vi "Expand.vi"(8 "error in (no error)":errorcluster, 9 "CurrentLinkedNodes":refnum<data-value>[](array[refnum]), 10 "NodeToExpand in":refnum<data-value>, 11 "OccupancyMap in":refnum<class "OccupancyMap.lvclass">) -> (0 "error out":errorcluster, 1 "NodesToLinkAndExpand":refnum<data-value>[](array[refnum]), 2 "NodeToExpand out":refnum<data-value>, 3 "OccupancyMap out":refnum<class "OccupancyMap.lvclass">)   [LabVIEW 2010, in "OccupancyMap.lvclass"]
uses:
  OccupancyMap.lvclass
  GraphNode/GraphNode.lvclass
  Cell/Cell.lvclass
  OccupancyMap.lvclass/OccupancyMap.ctl
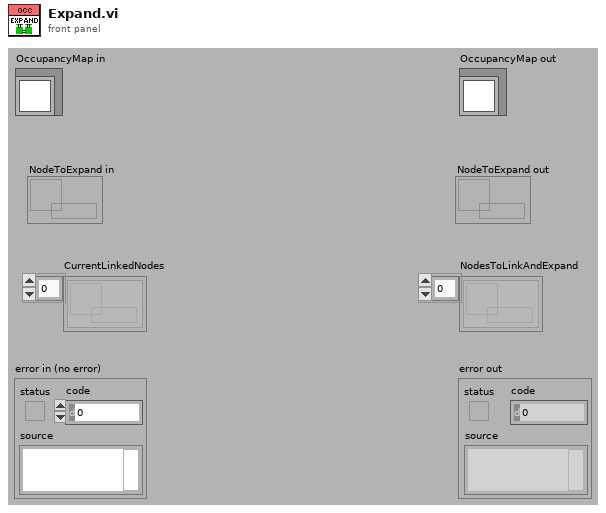
[diagram p1: front panel]
types:
  T1 = cluster{"Left":dbl, "Right":dbl, "Top":dbl, "Bottom":dbl}
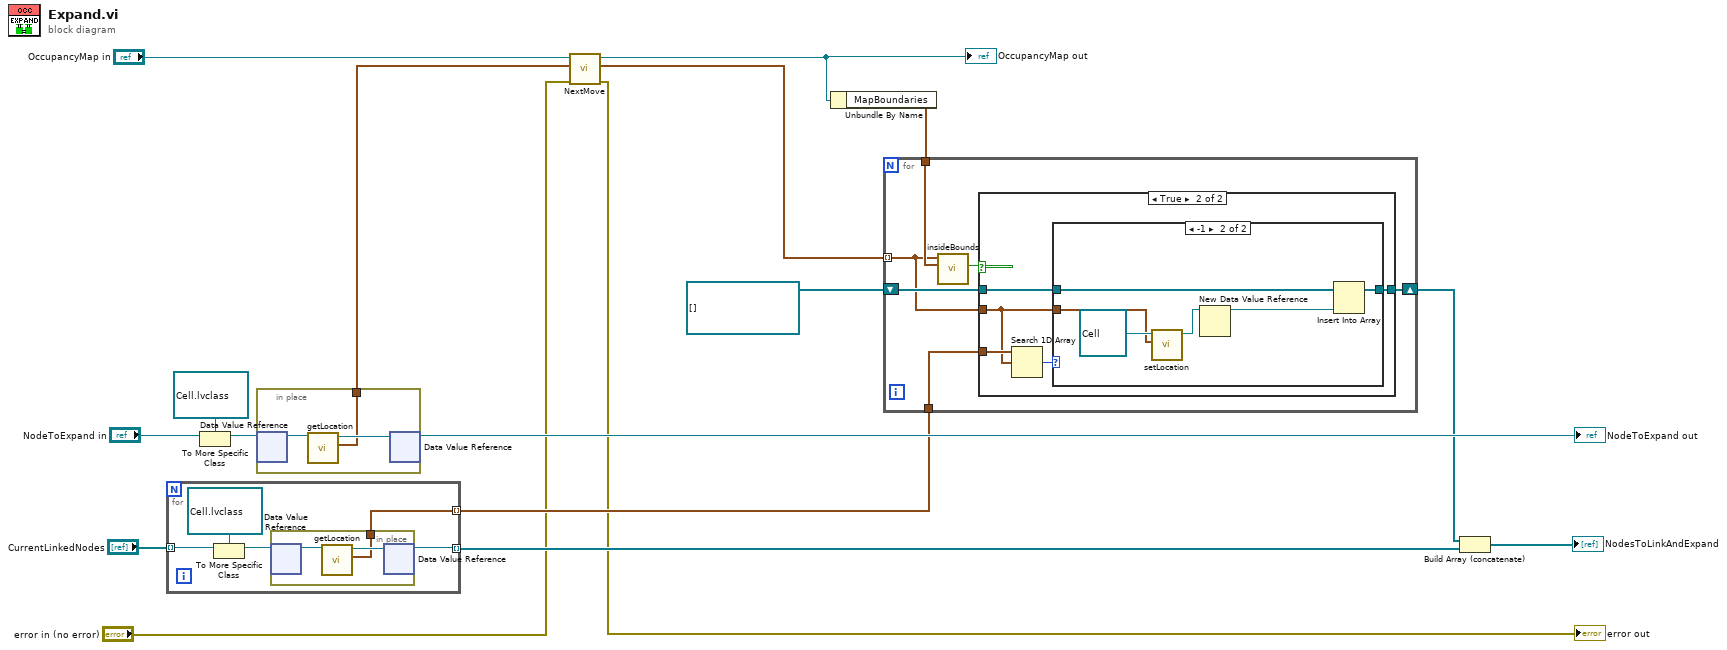
[diagram p0: block diagram]
diagram:
  n1 = for {
    tunnel: "CurrentLinkedNodes" -> [w20] mode=indexing
    tunnel: [w19] -> w11 mode=indexing
    tunnel: [w18] -> w8 mode=indexing
    n2 = To More Specific Class(target class=refnum<data-value> refnum ("data value reference"), reference=w20) -> (specific class reference=w22:refnum<data-value>)  [unwired: 1 in, 1 out]
    n3 = in-place {
      in-place-border: [w23] -> w19
      n4 = in-place-dvr #1(w22) -> (w25:refnum<class "Cell.lvclass">)  [unwired: 1 out]
      n5 = call "getLocation.vi"("Cell in"=w25) -> ("Location"=w23:cluster{"X":dbl, "Y":dbl}, "Cell out"=w24:refnum<class "Cell.lvclass">)  [unwired: 8 in, 1 out]
      n6 = in-place-dvr #1(w24) -> (w18:refnum<data-value>)  [unwired: 1 out]
    }
  }
  n7 = To More Specific Class(target class=refnum<data-value> refnum ("data value reference"), reference="NodeToExpand in") -> (specific class reference=w15:refnum<data-value>)  [unwired: 1 in, 1 out]
  n8 = in-place {
    in-place-border: [w26] -> w2
    n9 = in-place-dvr #2(w15) -> (w28:refnum<class "Cell.lvclass">)  [unwired: 1 out]
    n10 = call "getLocation.vi"("Cell in"=w28) -> ("Location"=w26:cluster{"X":dbl, "Y":dbl}, "Cell out"=w27:refnum<class "Cell.lvclass">)  [unwired: 8 in, 1 out]
    n11 = in-place-dvr #2(w27) -> (→"NodeToExpand out":refnum<data-value>)  [unwired: 1 out]
  }
  n12 = call "NextMove.vi"("error in (no error)"="error in (no error)", "Point"=w2, "OccupancyMap in"="OccupancyMap in") -> ("error out"=→"error out":errorcluster, "NextMove"=w1:cluster{"X":dbl, "Y":dbl}[], "OccupancyMap out"=w5:refnum<class "OccupancyMap.lvclass">)  [unwired: 6 in]
  "OccupancyMap out" <- w5
  n13 = Unbundle By Name(w5) -> ("MapBoundaries"=w12:T1)
  n14 = for {
    tunnel: w1 -> [w30] mode=indexing
    tunnel: w12 -> [w34]
    shift-right: [w32] -> w9
    shift-left: refnum<data-value>[] [] -> [w33]
    tunnel: w11 -> [w29]
    n15 = call "insideBounds.vi"("Rectangle"=w34, "point"=w30) -> ("inside"=w31:bool)  [unwired: 8 in, 1 out]
    n16 = case shown="True" w31 {
      tunnel: w33 -> [w35 w40]
      tunnel: [w35 w39] -> w32
      tunnel: w30 -> [_ w37]
      tunnel: w29 -> [_ w38]
      frame False {
      }
      frame True {
        n17 = Search 1D Array(1D array=w38, element=w37) -> (index of element=w36:i32)  [unwired: 1 in]
        n18 = case shown="-1" w36 {
          tunnel: w40 -> [w41 w47]
          tunnel: [w41 w46] -> w39
          tunnel: w37 -> [_ w44]
          frame Default {
          }
          frame -1 {
            n19 = call "setLocation.vi"("Location"=w44, "Cell in"=refnum<class "Cell.lvclass"> refnum ("Cell.lvclass")) -> ("Cell out"=w43:refnum<class "Cell.lvclass">)  [unwired: 8 in, 1 out]
            n20 = New Data Value Reference(data value=w43) -> (data value reference=w42:refnum<data-value>)  [unwired: 1 in, 1 out]
            n21 = Insert Into Array(array=w47, new element=w42) -> (w46:refnum<data-value>[])  [unwired: 1 in]
          }
        }
      }
    }
  }
  n22 = Build Array (concatenate)(w9, w8) -> (→"NodesToLinkAndExpand":refnum<data-value>[])
